vi "onListRequirements.vi"(8 "error in (no error)":errorcluster, 10 "Filter":T1, 11 "Pips.TestResults in":refnum<class "Pips.TestResults.lvclass">) -> (0 "error out":errorcluster, 2 "RequirementIDs":string[](array[string]), 3 "Pips.TestResults out":refnum<class "Pips.TestResults.lvclass">)   [LabVIEW 2021, in "Banana.Caraya.lvlib" / "Pips.TestResults.lvclass"]
uses:
  Pips.TestResults.lvclass
  Bananas/Pips/pip_filter -- enum.ctl
  Pips.TestResults.lvclass/Pips.TestResults.ctl
  Bananas/Pips/Pips.lvclass
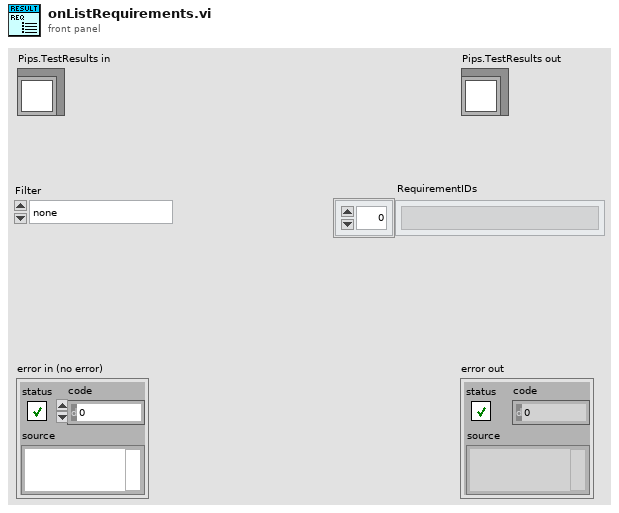
[diagram p1: front panel]
types:
  T1 = typedef "Bananas.lvlib/Pips.lvclass/pip_filter -- enum.ctl" = enum16{"none", "passed", "skipped", "covered", "uncovered"}
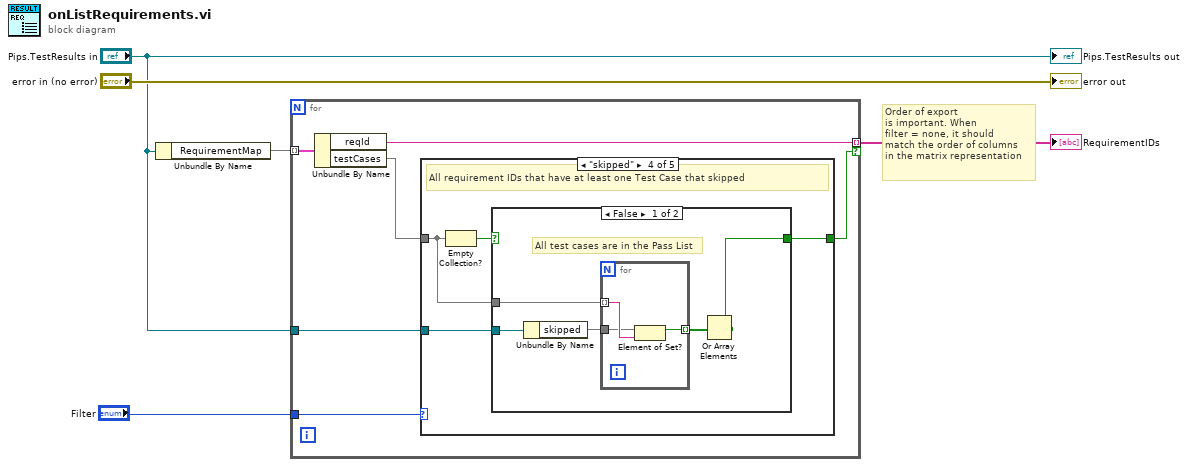
[diagram p0: block diagram]
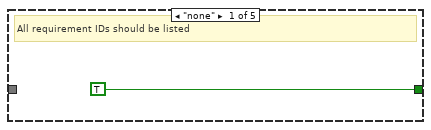
[diagram p2: hidden frame]
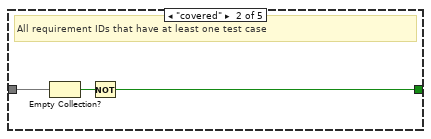
[diagram p3: hidden frame]
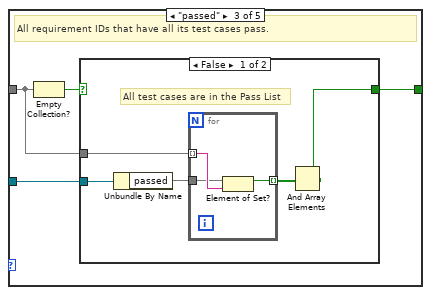
[diagram p4: hidden frame]
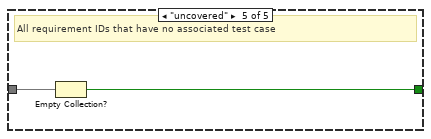
[diagram p7: hidden frame]
diagram:
  # "Order of export\nis important. When\nfilter = none, it should\nmatch the order of columns\nin the matrix representation"
  n1 = Unbundle By Name("Pips.TestResults in") -> ("RequirementMap"=w4:map{string, set{string}})
  n2 = for {
    tunnel: w4 -> [w11] mode=indexing
    tunnel: [w10] -> w3 mode=indexing if=w7
    tunnel: "Filter" -> [w9]
    tunnel: "Pips.TestResults in" -> [w6]
    n3 = Unbundle By Name(w11) -> ("reqId"=w10:string, "testCases"=w8:set{string})
    n4 = case shown="\"skipped\"" w9 {
      tunnel: w8 -> [_ w15 w17 w29 w41]
      tunnel: [TRUE w13 w18 w30 w40] -> w7
      tunnel: w6 -> [_ _ w16 w28 _]
      frame "none" {
        # "All requirement IDs should be listed"
      }
      frame "covered" {
        # "All requirement IDs that have at least one test case"
        n5 = Empty Collection?(1:w15) -> (0:w14:bool)
        n6 = Not(x=w14) -> (.not. x?=w13:bool)
      }
      frame "passed" {
        # "All requirement IDs that have all its test cases pass."
        n7 = Empty Collection?(1:w17) -> (0:w19:bool)
        n8 = case shown="False" w19 {
          tunnel: [w24 _] -> w18
          tunnel: w17 -> [w22 _]
          tunnel: w16 -> [w23 _]
          frame False {
            # "All test cases are in the Pass List"
            n9 = Unbundle By Name(w23) -> ("passed"=w21:set{string})
            n10 = for {
              tunnel: w22 -> [w27] mode=indexing
              tunnel: w21 -> [w26]
              tunnel: [w25] -> w20 mode=indexing
              n11 = Element of Set?(10:w27, 11:w26) -> (3:w25:bool)
            }
            n12 = And Array Elements(Boolean array=w20) -> (logical AND=w24:bool)
          }
          frame True {
          }
        }
      }
      frame "skipped" {
        # "All requirement IDs that have at least one Test Case that skipped"
        n13 = Empty Collection?(1:w29) -> (0:w31:bool)
        n14 = case shown="False" w31 {
          tunnel: [w36 _] -> w30
          tunnel: w29 -> [w34 _]
          tunnel: w28 -> [w35 _]
          frame False {
            # "All test cases are in the Pass List"
            n15 = Unbundle By Name(w35) -> ("skipped"=w33:set{string})
            n16 = for {
              tunnel: w34 -> [w39] mode=indexing
              tunnel: w33 -> [w38]
              tunnel: [w37] -> w32 mode=indexing
              n17 = Element of Set?(10:w39, 11:w38) -> (3:w37:bool)
            }
            n18 = Or Array Elements(Boolean array=w32) -> (logical OR=w36:bool)
          }
          frame True {
          }
        }
      }
      frame "uncovered" {
        # "All requirement IDs that have no associated test case"
        n19 = Empty Collection?(1:w41) -> (0:w40:bool)
      }
    }
  }
  "RequirementIDs" <- w3
  "error out" <- "error in (no error)"
  "Pips.TestResults out" <- "Pips.TestResults in"
